vi "Read Input Graph.vi"(8 "error in (no error)":errorcluster, 11 "AbstractExtractor1D in":refnum<class "AbstractExtractor1D.lvclass">) -> (0 "error out":errorcluster, 2 "Input Graph":refnum<vi>, 3 "AbstractExtractor1D out":refnum<class "AbstractExtractor1D.lvclass">)   [LabVIEW 2014]
uses:
  AbstractExtractor1D.lvclass
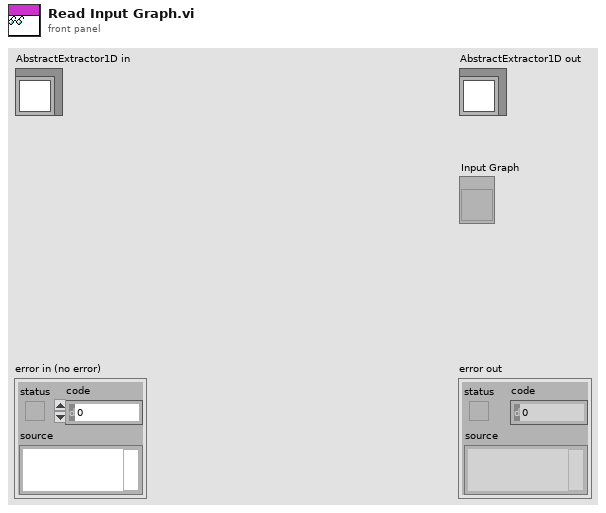
[diagram p1: front panel]
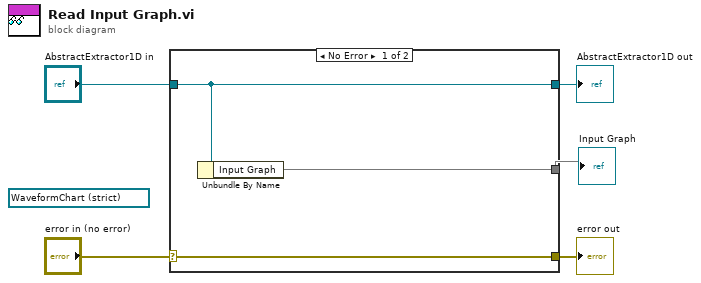
[diagram p0: block diagram]
diagram:
  (unwired) refnum<vi> refnum ("Result Graph")
  n1 = case shown="No Error" "error in (no error)" {
    selector: "error in (no error)" -> [w8 w9]
    tunnel: [w8 w9] -> w4
    tunnel: [w7 w10] -> w2
    tunnel: "AbstractExtractor1D in" -> [w7 w10]
    tunnel: [w6 _] -> w1
    frame No Error {
      n2 = Unbundle By Name(w7) -> ("Input Graph"=w6)
    }
    frame Error {
    }
  }
  "error out" <- w4
  "AbstractExtractor1D out" <- w2
  "Input Graph" <- w1
